vi "Check Connection to a Real-Time System LV2012 NIVerified.vi"() -> ()   [LabVIEW 2012]
doc: "This VI demonstrates how to check, if a Real-Time system is available in the network or not.\n<b>Please keep in mind, that the VI used in this example is deprecated since LabVIEW Real-Time 2012.<b>\nUse the System Configuration API instead."
uses:
  <vilib>/real-time/rtutility.llb/RT Get Target Information (IP).vi
  <vilib>/real-time/NI_Real-Time Libraries.lvlib
panel:
  out "Connection Status":string
  in  "Target Address":string="10.0.35.206"
  # "Overview: Demonstrates how to programmatically check if a Real-Time system is connected to the network or not. \nRequirements: LabVIEW Base Development System 2012 (or compatible)\n                             LabVIEW Real-Time Module 2012 (or compatible)\nInstructions: \n1. Enter the IP address or DNS name of the target.\n2. Run the VI."
  # "Note\nPlease keep in mind, that the VI used in this example is deprecated since LabVIEW Real-Time 2012.\nUse the System Configuration API instead."
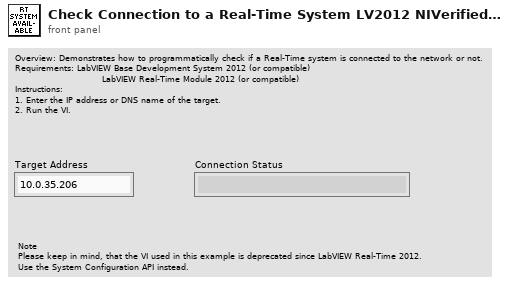
[diagram p1: front panel]
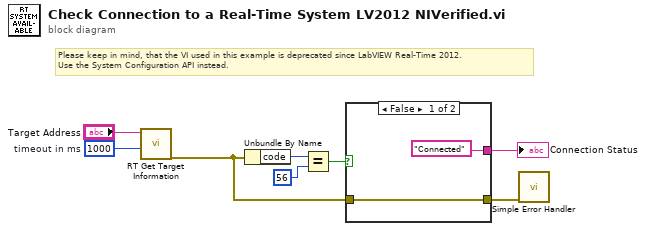
[diagram p0: block diagram]
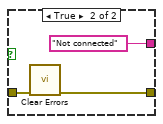
[diagram p2: hidden frame]
diagram:
  w2 = 1000  # timeout in ms
  # "Please keep in mind, that the VI used in this example is deprecated since LabVIEW Real-Time 2012.\nUse the System Configuration API instead."
  n1 = call-poly <vilib>:"RT Get Target Information.vi"("timeout in ms (10000)"=w2, "target address"="Target Address") -> ("error out"=w4:errorcluster)  [unwired: 8 in, 1 out]
  n2 = Unbundle By Name(w4) -> ("code"=w7:i32)
  n3 = Equal?(x=w7, y=56) -> (x = y?=w5:bool)
  n4 = case shown="False" w5 {
    tunnel: w4 -> [w9 w13]
    tunnel: ["Connected" "Not connected"] -> w3
    tunnel: [w9 w11] -> w1
    frame False {
    }
    frame True {
      n5 = call <vilib>:"Clear Errors.vi"("error in (no error)"=w13) -> ("error out"=w11:errorcluster)  [unwired: 6 in]
    }
  }
  "Connection Status" <- w3
  n6 = call <vilib>:"Simple Error Handler.vi"("error in (no error)"=w1) -> ()  [unwired: 4 in, 5 out]
